vi "Assemble BoundViewManager.vi"(4 "Default View Name (\"\"=None)":string, 6 "Startup View Name (\"\"=None)":string, 7 "Insert View on Value Change Only? (T)":bool=TRUE, 8 "Selector String Name":string, 9 "Viewable Names":string[](array[string]), 10 "Bound Viewables":refnum<class "IViewable.lvclass">[](array[class])) -> (3 "BoundViewManager Out":refnum<class "BoundViewManager.lvclass">)   [LabVIEW 2017, in "BoundViewManager.lvlib" / "BoundViewManager.lvclass"]
doc: "<License>\nCopyright © 2017 Composed Systems, LLC | All rights reserved\nwww.composed.io\n\nAuthor: Ethan Stern <ethan.stern@composed.io>\n\nThis software is provided \"AS IS\" WITHOUT WARRANTIES, either express or implied, AND IS FOR EDUCATIONAL PURPOSES ONLY.\n</License>"
uses:
  BoundViewManager.lvclass
  C:/Git/mva-framework/Framework/IViewManager/IViewManager/IViewManager.lvclass
  Framework/IViewable/IViewable/IViewable.lvclass
  Framework/IViewManager/IViewManager Messages/Launch Nested Views Msg/Launch Nested Views Msg.lvclass/Launch Nested Views Msg.ctl
  Framework/IViewManager/IViewManager/IViewManager.lvclass/IViewManager.ctl
  BoundViewManager.lvclass/BoundViewManager.ctl
  Framework/IViewManager/IViewManager Messages/Launch Nested Views Msg/Pack Launch Nested Views Msg.vi
  Framework/IViewManager/IViewManager Messages/Launch Nested Views Msg/Launch Nested Views Msg.lvclass
  Framework/IViewManager/IViewManager/IViewManager.lvclass
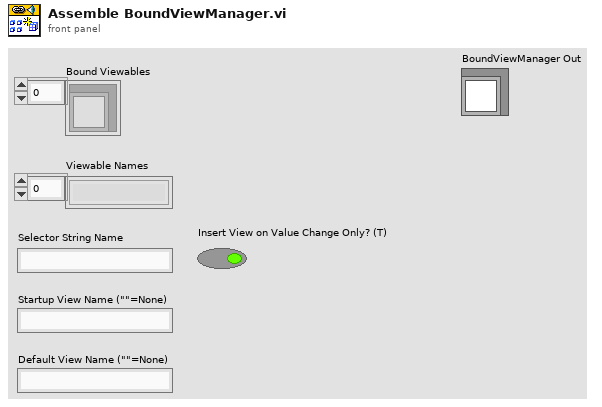
[diagram p1: front panel]
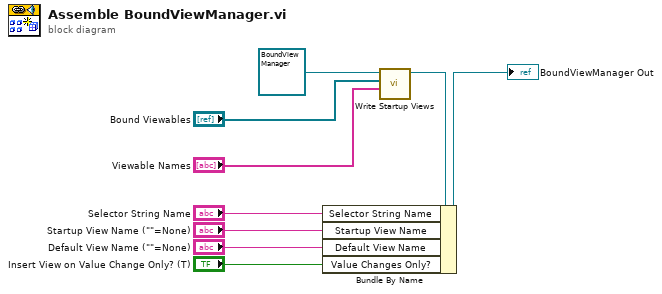
[diagram p0: block diagram]
diagram:
  n1 = call "Write Startup Views.vi"("View Labels"="Viewable Names", "Startup Views"="Bound Viewables", "IViewManager in"=refnum<class "BoundViewManager.lvclass"> refnum ("BoundViewManager")) -> ("IViewManager out"=w6:refnum<class "BoundViewManager.lvclass">)  [unwired: 8 in]
  n2 = Bundle By Name(cluster=w6, "Selector String Name"="Selector String Name", "Startup View Name"="Startup View Name (\"\"=None)", "Default View Name"="Default View Name (\"\"=None)", "Value Changes Only?"="Insert View on Value Change Only? (T)") -> (→"BoundViewManager Out":refnum<class "BoundViewManager.lvclass">)
